vi "Daten Serialisieren - GPS.vi"(6 "GPS Position":sgl[](array[numeric]), 9 "Frame-ID":u32, 10 "Aktuelle Zeit":timestamp, 11 "GPS Datum & Zeit":sgl[](array[numeric])) -> (2 "data":T1[](array[typedef])=[{"timestamp"=timestamp(0 s since 1904-01-01), "payload"=[0, 2, 3, 4, 5, 6, 7, 8], "identifier"=2, "type"=0, "extended?"=FALSE, "echo?"=FALSE}, {"timestamp"=timestamp(0 s since 1904-01-01), "payload"=[0, 1, 2, 3, 4, 5, 6, 7], "identifier"=3, "type"=0, "extended?"=FALSE, "echo?"=FALSE}] {"payload" format="%x"; "timestamp" format="%<%.7X\n%x>T"; "type" items=["CAN Data"=0, "CAN Remote"=1, "CAN Bus Error"=2, "CAN 2.0 Data"=8, "CAN FD Data"=16, "CAN FD+BRS Data"=24, "J1939 Data"=192, "Delay"=224, "Log Trigger"=225, "Start Trigger"=226]; "identifier" format="%x"})   [LabVIEW 2020, in "CAN Interface.lvlib"]
uses:
  CAN Interface.lvlib
  <vilib>/xnet/xnet.llb/XNET Frame CAN.ctl
  <vilib>/xnet/xnet.llb/XNET Frame Type CAN.ctl
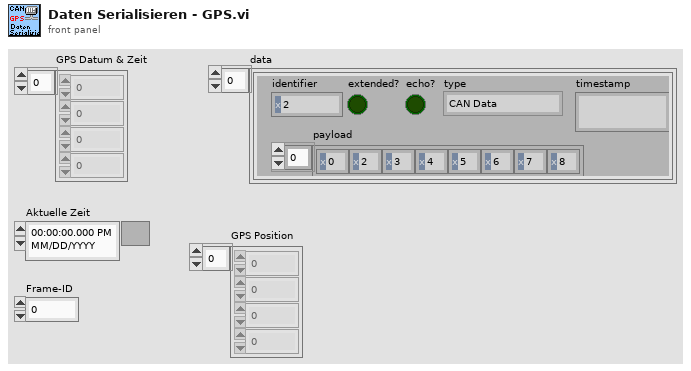
[diagram p1: front panel]
types:
  T1 = typedef "XNET Frame CAN.ctl" = cluster{"timestamp":timestamp, "payload":u8[], "identifier":u32, "type":T2, "extended?":bool, "echo?":bool}
  T2 = typedef "XNET Frame Type CAN.ctl" = u8
  T3 = enum16{"big-endian, network order", "native, host order", "little-endian"}
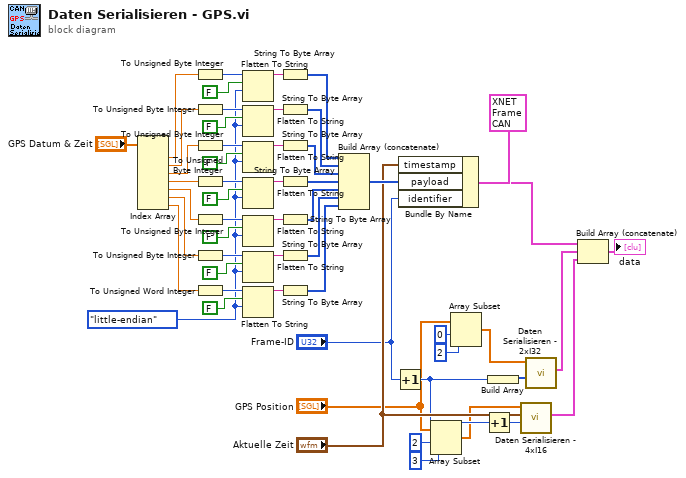
[diagram p0: block diagram]
diagram:
  w25 = T3."little-endian" ("Byte-Reihenfolge (0:Big-Endian, Netzwerkreihenfolge)")
  n1 = Index Array(array="GPS Datum & Zeit") -> (element #1=w20:sgl, element #2=w19:sgl, element #3=w18:sgl, element #4=w17:sgl, element #5=w16:sgl, element #6=w15:sgl, element #7=w14:sgl)  [unwired: 7 in]
  n2 = To Unsigned Byte Integer(number=w20) -> (unsigned 8bit integer=w53:u8)
  n3 = To Unsigned Byte Integer(number=w19) -> (unsigned 8bit integer=w52:u8)
  n4 = To Unsigned Byte Integer(number=w18) -> (unsigned 8bit integer=w47:u8)
  n5 = To Unsigned Byte Integer(number=w17) -> (unsigned 8bit integer=w46:u8)
  n6 = To Unsigned Byte Integer(number=w16) -> (unsigned 8bit integer=w41:u8)
  n7 = To Unsigned Byte Integer(number=w15) -> (unsigned 8bit integer=w40:u8)
  n8 = To Unsigned Word Integer(number=w14) -> (unsigned 16bit integer=w35:u16)
  n9 = Flatten To String(anything=w53, prepend array or string size? (T)=FALSE ("Array- oder String-Größe voranstellen? (T)"), byte order (0:big-endian, network order)=w25) -> (data string=w55:string)  [unwired: 1 in, 2 out]
  n10 = Flatten To String(anything=w52, prepend array or string size? (T)=FALSE ("Array- oder String-Größe voranstellen? (T)"), byte order (0:big-endian, network order)=w25) -> (data string=w50:string)  [unwired: 1 in, 2 out]
  n11 = Flatten To String(anything=w47, prepend array or string size? (T)=FALSE ("Array- oder String-Größe voranstellen? (T)"), byte order (0:big-endian, network order)=w25) -> (data string=w49:string)  [unwired: 1 in, 2 out]
  n12 = Flatten To String(anything=w46, prepend array or string size? (T)=FALSE ("Array- oder String-Größe voranstellen? (T)"), byte order (0:big-endian, network order)=w25) -> (data string=w44:string)  [unwired: 1 in, 2 out]
  n13 = Flatten To String(anything=w41, prepend array or string size? (T)=FALSE ("Array- oder String-Größe voranstellen? (T)"), byte order (0:big-endian, network order)=w25) -> (data string=w43:string)  [unwired: 1 in, 2 out]
  n14 = Flatten To String(anything=w40, prepend array or string size? (T)=FALSE ("Array- oder String-Größe voranstellen? (T)"), byte order (0:big-endian, network order)=w25) -> (data string=w38:string)  [unwired: 1 in, 2 out]
  n15 = Flatten To String(anything=w35, prepend array or string size? (T)=FALSE ("Array- oder String-Größe voranstellen? (T)"), byte order (0:big-endian, network order)=w25) -> (data string=w37:string)  [unwired: 1 in, 2 out]
  n16 = String To Byte Array(string=w55) -> (unsigned byte array=w34:u8[])
  n17 = String To Byte Array(string=w50) -> (unsigned byte array=w33:u8[])
  n18 = String To Byte Array(string=w49) -> (unsigned byte array=w32:u8[])
  n19 = String To Byte Array(string=w44) -> (unsigned byte array=w31:u8[])
  n20 = String To Byte Array(string=w43) -> (unsigned byte array=w30:u8[])
  n21 = String To Byte Array(string=w38) -> (unsigned byte array=w29:u8[])
  n22 = String To Byte Array(string=w37) -> (unsigned byte array=w28:u8[])
  n23 = Build Array (concatenate)(w34, w33, w32, w31, w30, w29, w28) -> (w27:u8[])
  n24 = Increment(x="Frame-ID") -> (x+1=w8:u32)
  n25 = Bundle By Name(cluster=T1 {"timestamp"=timestamp(0 s since 1904-01-01), "payload"=[0, 2, 3, 4, 5, 6, 7, 8], "identifier"=2, "type"=0, "extended?"=FALSE, "echo?"=FALSE} ("CAN frame"), "timestamp"="Aktuelle Zeit", "payload"=w27, "identifier"="Frame-ID") -> (w23:T1)
  n26 = Array Subset(array="GPS Position", index=2 ("Index"), length=3 ("Länge")) -> (w1:sgl[])
  n27 = Array Subset(array="GPS Position", index=0 ("Index"), length=2 ("Länge")) -> (w7:sgl[])
  n28 = Increment(x=w8) -> (x+1=w11:u32)
  n29 = Build Array(w8) -> (w9:u32[])
  n30 = call "Daten Serialisieren - 4xI16.vi"("Frame-ID"=w11, "Aktuelle Zeit"="Aktuelle Zeit", "Messdaten"=w1) -> ("data"=w13:T1[])  [unwired: 7 in, 1 out]
  n31 = call "Daten Serialisieren - 2xI32.vi"("Frame-ID"=w9, "Messdaten"=w7) -> ("data"=w12:T1[])  [unwired: 9 in]
  n32 = Build Array (concatenate)(w23, w12, w13) -> (→"data":T1[])
